vi "DrawOGLText.vi"(0 "Text":T1={"Text"="", "Color Box"=10395294, "Alpha"=1.0, "Font file"=path "/Volumes/Kim/Library/Fonts/Tahoma.ttf"}, 1 "Name":string, 3 "error in (no error)":errorcluster) -> (5 "object out":refnum<vi>, 7 "error out":errorcluster)   [LabVIEW 2017]
uses:
  <vilib>/picture/3D Picture Control/Object/Create Object (name).vi
  <vilib>/picture/3D Picture Control/NI_3D Picture Control.lvlib
panel:
  out "Color":T2={"Red"=1.0, "Green"=0.0, "Blue"=0.0, "Alpha"=1.0}
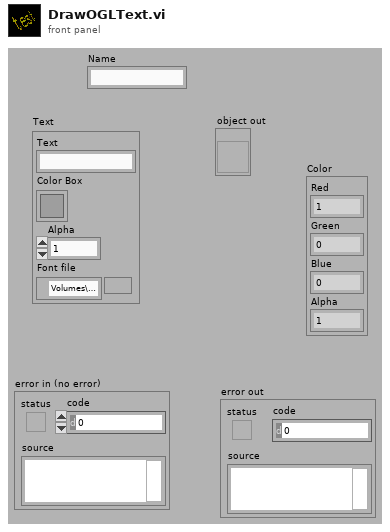
[diagram p1: front panel]
types:
  T1 = cluster{"Text":string, "Color Box":u32, "Alpha":sgl, "Font file":path}
  T2 = cluster{"Red":sgl, "Green":sgl, "Blue":sgl, "Alpha":sgl}
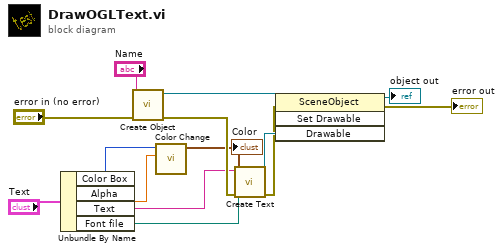
[diagram p0: block diagram]
diagram:
  n1 = Unbundle By Name("Text") -> ("Color Box"=w7:u32, "Alpha"=w6:sgl, "Text"=w2:string, "Font file"=w1:path)
  n2 = call-poly <vilib>:"Create Object.vi"("error in (no error)"="error in (no error)", "Name"="Name") -> ("error out"=w9:errorcluster, "Scene:New Object"=w12:refnum<vi>)  [unwired: 8 in]
  n3 = call <vilib>:"Color Change.vi"("Alpha"=w6, "Color"=w7) -> ("RGBA"=w5:cluster{"R":sgl, "G":sgl, "B":sgl, "A":sgl})  [unwired: 9 in]
  "Color" <- w5
  n4 = call <vilib>:"Create Text.vi"("error in (no error)"=w9, "Color"=w5, "Path to font file"=w1, "Text"=w2) -> ("error out"=w8:errorcluster, "New Text Refnum"=w13:refnum<vi>)  [unwired: 6 in]
  n5 = invoke class="SceneObject" method="Set Drawable"(reference=w12, error in=w8, "Drawable"=w13) -> (reference out=→"object out":refnum<vi>, error out=→"error out":errorcluster)  [unwired: 1 in, 2 out]
